vi "Abort.Send Abort or Done Notificaiton.vi"(7 "Abort Notifier Name":string="Abort", 10 "Error":errorcluster, 11 "Abort(T)/Done(F)":bool) -> (2 "error out":errorcluster)   [LabVIEW 2018]
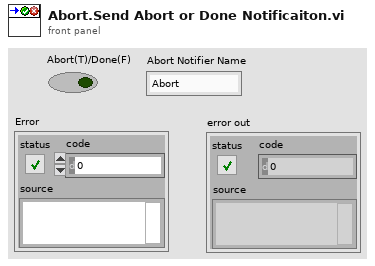
[diagram p1: front panel]
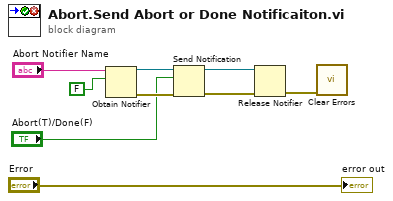
[diagram p0: block diagram]
diagram:
  n1 = Obtain Notifier(name (unnamed)="Abort Notifier Name", notification data type=FALSE) -> (notifier out=w7:refnum<notifier>, error out=w6:errorcluster)  [unwired: 2 in, 1 out]
  n2 = Send Notification(notification="Abort(T)/Done(F)", notifier=w7, error in (no error)=w6) -> (notifier out=w4:refnum<notifier>, error out=w5:errorcluster)
  n3 = Release Notifier(notifier=w4, error in (no error)=w5) -> (error out=w3:errorcluster)  [unwired: 1 in, 2 out]
  n4 = call <vilib>:"Clear Errors.vi"("error in (no error)"=w3) -> ()  [unwired: 5 in, 2 out]
  "error out" <- "Error"
